vi "Driving Encoder Distance.vi"(8 "Speed":dbl, 9 "Use Distance?":bool, 10 "Setpoint Angle":dbl, 11 "Setpoint Distance":dbl) -> (1 "PID Data":T1, 2 "Motor Output":dbl, 3 "Gyro Angle":dbl)   [LabVIEW 2014]
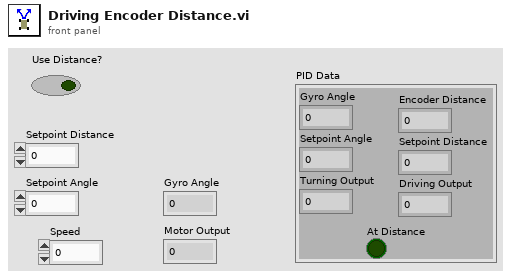
[diagram p1: front panel]
types:
  T1 = cluster{"Gyro Angle":dbl, "Setpoint Angle":dbl, "Turning Output":dbl, dbl, "Setpoint Distance":dbl, "Driving Output":dbl, bool}
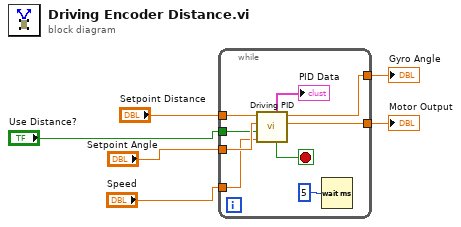
[diagram p0: block diagram]
diagram:
  n1 = while {
    tunnel: "Setpoint Distance" -> [w11]
    tunnel: "Setpoint Angle" -> [w10]
    tunnel: [w14] -> w4
    tunnel: [w13] -> w3
    tunnel: "Use Distance?" -> [w8]
    tunnel: "Speed" -> [w7]
    stop <- w12 stop-if-true
    n2 = call "Driving PID.vi"("Manual Speed"=w7, "Use Distance?"=w8, "Setpoint Angle"=w10, "Setpoint Distance"=w11) -> ("Turning Output"=w13:dbl, "Gyro Angle"=w14:dbl, "Boolean Output"=w12:bool, "PID Data"=→"PID Data":T1)  [unwired: 2 in, 2 out]
    n3 = Wait (ms)(milliseconds to wait=u32 5) -> ()  [unwired: 1 out]
  }
  "Motor Output" <- w3
  "Gyro Angle" <- w4
